vi "Function.vi"   [LabVIEW 2016]
uses:
  <vilib>/NXT/Hardware/Plugins/Tetrix 180 deg Servo/Tetrix180ServoAddress.ctl
  <vilib>/NXT/NXTIO Xnodes/NXTIONodeSubVIs/TETRIX IO Move Servos.vi
  <vilib>/NXT/Dual Mode Library/Waits/Wait_Num.vi
  <vilib>/NXT/NXTIO Xnodes/AddressXNode/NXTIOAddress.xnode
  <vilib>/NXT/Subs/LVHSConnector.ctl
  <vilib>/NXT/NXTIO Xnodes/NXTIOXNode/NXTIO.xnode
  <vilib>/NXT/LegoClasses/BrickReference/BrickReference.lvclass
types:
  T1 = typedef "Tetrix180ServoAddress.ctl" = i32
  T2 = cluster{"Tetrix180Servo":T1, "Tetrix180Servo":T1}
  T3 = typedef "LVHSConnector.ctl" = refnum<class "BrickReference.lvclass">
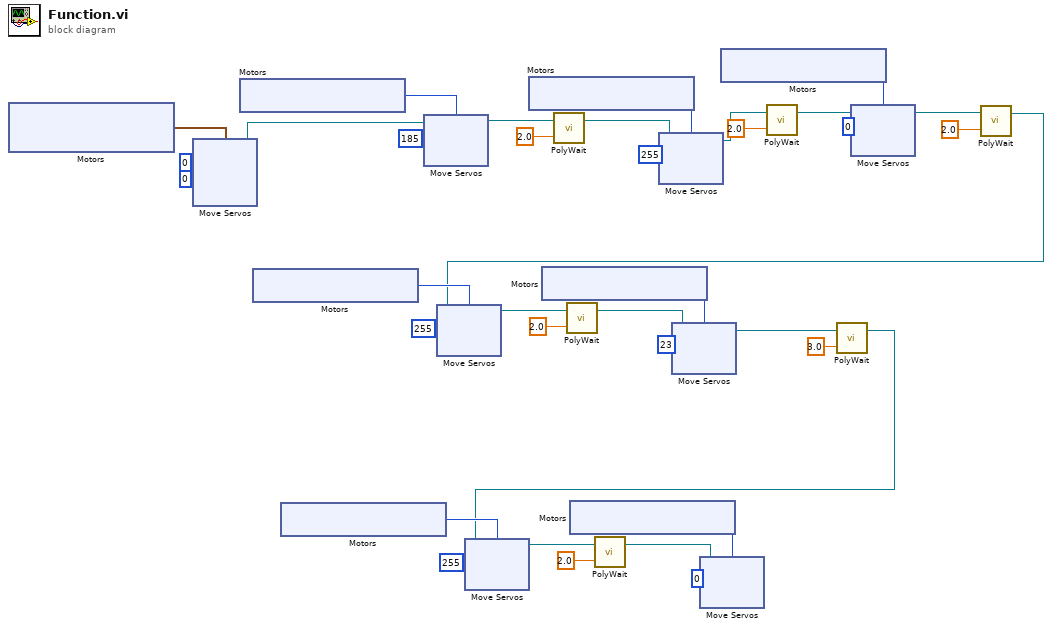
[diagram p0: block diagram]
diagram:
  n1 = xnode "Motors"() -> ("Motor"=w3:T2)
  n2 = xnode "Move Servos"("Position 2"=u8 0, "Position 1"=u8 0, "Motors"=w3) -> ("NXT/EV3"=w2:T3)  [unwired: 1 in]
  n3 = xnode "Motors"() -> ("Motor"=w36:T1)
  n4 = xnode "Motors"() -> ("Motor"=w18:T1)
  n5 = xnode "Motors"() -> ("Motor"=w13:T1)
  n6 = xnode "Move Servos"("Position 1"=u8 185, "Motors"=w36, "NXT/EV3"=w2) -> ("NXT/EV3"=w34:T3)
  n7 = xnode "Motors"() -> ("Motor"=w32:T1)
  n8 = xnode "Motors"() -> ("Motor"=w22:T1)
  n9 = call-poly <vilib>:"PolyWait.vi"("Time (1 sec)"=sgl 2.0, "NXT/EV3"=w34) -> ("NXT/EV3"=w31:T3)  [unwired: 2 in]
  n10 = xnode "Motors"() -> ("Motor"=w9:T1)
  n11 = xnode "Move Servos"("Position 1"=u8 255, "Motors"=w32, "NXT/EV3"=w31) -> ("NXT/EV3"=w27:T3)
  n12 = xnode "Motors"() -> ("Motor"=w29:T1)
  n13 = call-poly <vilib>:"PolyWait.vi"("Time (1 sec)"=sgl 2.0, "NXT/EV3"=w27) -> ("NXT/EV3"=w25:T3)  [unwired: 2 in]
  n14 = xnode "Move Servos"("Position 1"=u8 0, "Motors"=w29, "NXT/EV3"=w25) -> ("NXT/EV3"=w16:T3)
  n15 = call-poly <vilib>:"PolyWait.vi"("Time (1 sec)"=sgl 2.0, "NXT/EV3"=w16) -> ("NXT/EV3"=w5:T3)  [unwired: 2 in]
  n16 = xnode "Move Servos"("Position 1"=u8 255, "Motors"=w18, "NXT/EV3"=w5) -> ("NXT/EV3"=w20:T3)
  n17 = call-poly <vilib>:"PolyWait.vi"("Time (1 sec)"=sgl 2.0, "NXT/EV3"=w20) -> ("NXT/EV3"=w23:T3)  [unwired: 2 in]
  n18 = xnode "Move Servos"("Position 1"=u8 23, "Motors"=w22, "NXT/EV3"=w23) -> ("NXT/EV3"=w15:T3)
  n19 = call-poly <vilib>:"PolyWait.vi"("Time (1 sec)"=sgl 3.0, "NXT/EV3"=w15) -> ("NXT/EV3"=w6:T3)  [unwired: 2 in]
  n20 = xnode "Move Servos"("Position 1"=u8 255, "Motors"=w13, "NXT/EV3"=w6) -> ("NXT/EV3"=w11:T3)
  n21 = call-poly <vilib>:"PolyWait.vi"("Time (1 sec)"=sgl 2.0, "NXT/EV3"=w11) -> ("NXT/EV3"=w8:T3)  [unwired: 2 in]
  n22 = xnode "Move Servos"("Position 1"=u8 0, "Motors"=w9, "NXT/EV3"=w8) -> ()  [unwired: 1 out]
